vi "Swerve_Module Drive Read Config.vi"(6 "Send Cmd Timout(ms)":u32=300, 8 "Error":errorcluster, 10 "Module Drive Config Data":T1={"ModuleDrive Ver"=0, "Output"={"Type"=enum."Counter-Clockwise", "Neutral"=enum."EEPROMSetting", "Max"={"FWD"=0.0, "REV"=0.04}, "Min"={"FWD"=0.0, "REV"=0.0}, "OL Ramp Rate (S)"=0.0, "Dead Band"=0.0}, "CL"={"Gains"={"P"=1.0, "I"=0.01, "D"=0.0, "F"=0.0}, "Error Allowed"={"High"=0.0, "Low"=0.0}, "I Zone"={"High"=10000.0, "Low"=-1000.0}, "Max Out"={"FWD"=1.0, "REV"=-1.0}, "Max I Accu"={"High"=10.0, "Low"=-10.0}, "CL Ramp Rate (S)"=0.0}, "VoltageComp"={"Enable"=FALSE, "Value"=0.0}} {"Output"."Min"."REV" format="%.2f"; "Output"."Min"."FWD" format="%.2f"; "Output"."Max"."REV" format="%.2f"; "Output"."Max"."FWD" format="%.2f"; "VoltageComp"."Value" format="%.1g"; "CL"."Max I Accu"."Low" format="%#.8f"; "CL"."Max I Accu"."High" format="%#.8f"; "CL"."Gains"."F" format="%#.8f"; "CL"."Gains"."D" format="%#.8f"; "CL"."Gains"."I" format="%#.8f"; "CL"."Gains"."P" format="%#.8f"; "CL"."Error Allowed"."Low" format="%#.8f"; "CL"."Error Allowed"."High" format="%#.8f"; "CL"."I Zone"."Low" format="%#.8f"; "CL"."I Zone"."High" format="%#.8f"; "CL"."Max Out"."REV" format="%.2f"; "CL"."Max Out"."FWD" format="%.2f"}, 11 "PhoenixMotorControlDevRef":T10={"DeviceStatus"={"status"=FALSE, "code"=0, "source"=""}, "Type"=enum."PWM", "PWM"={"PWM Channel"=enum."Invalid", "DeadBand"={"Name"="", "maxPositivePwm"=0, "minPositivePwm"=0, "centerPwm"=0, "maxNegativePwm"=0, "minNegativePwm"=0, "angularRange"=0}}, "CAN"={"Device Number"=0, "SetOutput VI Ref"=variant, "GetOutput VI Ref"=variant, "Enable VI Ref"=variant, "Disable VI Ref"=variant, "Data"=variant}, "Invert"=FALSE, "DIO PWM"={"PWM \"Enable\" Channel"=enum."Invalid", "DIOChannel"=enum."Invalid", "PWM Rate"=0.0}}) -> (0 "Error Out":errorcluster, 2 "Module Azimuth Config Data Out":T1={"ModuleDrive Ver"=0, "Output"={"Type"=enum."Counter-Clockwise", "Neutral"=enum."EEPROMSetting", "Max"={"FWD"=0.0, "REV"=0.04}, "Min"={"FWD"=0.0, "REV"=0.0}, "OL Ramp Rate (S)"=0.0, "Dead Band"=0.0}, "CL"={"Gains"={"P"=1.0, "I"=0.01, "D"=0.0, "F"=0.0}, "Error Allowed"={"High"=0.0, "Low"=0.0}, "I Zone"={"High"=10000.0, "Low"=-1000.0}, "Max Out"={"FWD"=1.0, "REV"=-1.0}, "Max I Accu"={"High"=10.0, "Low"=-10.0}, "CL Ramp Rate (S)"=0.0}, "VoltageComp"={"Enable"=FALSE, "Value"=0.0}} {"Output"."Min"."REV" format="%.2f"; "Output"."Min"."FWD" format="%.2f"; "Output"."Max"."REV" format="%.2f"; "Output"."Max"."FWD" format="%.2f"; "VoltageComp"."Value" format="%.1g"; "CL"."Max I Accu"."Low" format="%#.8f"; "CL"."Max I Accu"."High" format="%#.8f"; "CL"."Gains"."F" format="%#.8f"; "CL"."Gains"."D" format="%#.8f"; "CL"."Gains"."I" format="%#.8f"; "CL"."Gains"."P" format="%#.8f"; "CL"."Error Allowed"."Low" format="%#.8f"; "CL"."Error Allowed"."High" format="%#.8f"; "CL"."I Zone"."Low" format="%#.8f"; "CL"."I Zone"."High" format="%#.8f"; "CL"."Max Out"."REV" format="%.2f"; "CL"."Max Out"."FWD" format="%.2f"}, 3 "Module Azimuth Ref Out":T10)   [LabVIEW 2023]
uses:
  <vilib>/Utility/Data Type/NI_Data Type.lvlib
  <vilib>/Rock Robotics/WPI/ThirdParty/Phoenix-LabVIEW/Motor Controller/Controls/CTRE_Phoenix_MotorControl_RemoteSourceType.ctl
  <vilib>/Rock Robotics/WPI/ThirdParty/Phoenix-LabVIEW/Motor Controller/Controls/CTRE_Phoenix_MotorControl_FeedbackDevice_TalonFX.ctl
  <vilib>/Rock Robotics/WPI/ThirdParty/Phoenix-LabVIEW/Motor Controller/Controls/CTRE_Phoenix_MotorControl_NeutralMode.ctl
  <vilib>/Rock Robotics/WPI/ThirdParty/Phoenix-LabVIEW/Motor Controller/Controls/CTRE_Phoenix_MotorControl_VelocityMeasurementPeriod.ctl
  <vilib>/Rock Robotics/WPI/ThirdParty/Phoenix-LabVIEW/Motor Controller/Controls/CTRE_Phoenix_MotorControl_SlotStructure.ctl
  <vilib>/Rock Robotics/WPI/ThirdParty/Phoenix-LabVIEW/Motor Controller/Controls/CTRE_Phoenix_MotorControl_FilterStruct.ctl
  <vilib>/Rock Robotics/WPI/ThirdParty/Phoenix-LabVIEW/Controls/CTRE_Phoenix_CustomParamConfiguration.ctl
  <vilib>/Rock Robotics/WPI/ThirdParty/Phoenix-LabVIEW/Motor Controller/Controls/CTRE_Phoenix_MotorControl_BaseConfigurables.ctl
  <vilib>/Rock Robotics/WPI/ThirdParty/Phoenix-LabVIEW/Motor Controller/Controls/CTRE_Phoenix_MotorControl_LimitSwitchNormal.ctl
  <vilib>/Rock Robotics/WPI/ThirdParty/Phoenix-LabVIEW/Motor Controller/Controls/CTRE_Phoenix_MotorControl_LimitSwitchSource_Local.ctl
  <vilib>/Rock Robotics/WPI/ThirdParty/Phoenix-LabVIEW/Motor Controller/Controls/CTRE_Phoenix_MotorControl_SupplyCurrentLimitConfiguration.ctl
  <vilib>/Rock Robotics/WPI/ThirdParty/Phoenix-LabVIEW/Motor Controller/Controls/CTRE_Phoenix_MotorControl_StatorCurrentLimitConfiguration.ctl
  <vilib>/Rock Robotics/WPI/ThirdParty/Phoenix-LabVIEW/Motor Controller/Controls/CTRE_Phoenix_MotorControl_MotorCommutation_TalonFX.ctl
  <vilib>/Rock Robotics/WPI/ThirdParty/Phoenix-LabVIEW/CANCoder/Controls/CTRE_Phoenix_CANcoder_AbsoluteSensorRange.ctl
  <vilib>/Rock Robotics/WPI/ThirdParty/Phoenix-LabVIEW/CANCoder/Controls/CTRE_Phoenix_CANcoder_SensorInitializationStrategy.ctl
  <vilib>/Rock Robotics/WPI/ThirdParty/Phoenix-LabVIEW/Motor Controller/Controls/CTRE_Phoenix_MotorControl_TalonFXMotorControllerConfigurables.ctl
  <vilib>/Rock Robotics/WPI/ThirdParty/Phoenix-LabVIEW/Motor Controller/Controls/CTRE_Phoenix_MotorControl_TalonFXInvertType.ctl
  <vilib>/Rock Robotics/SystemInterfaces/DIO/FPGA_DIOPWMChannel.ctl
  <vilib>/Rock Robotics/WPI/PWM/WPI_PWMDeadband.ctl
  <vilib>/Rock Robotics/WPI/MotorControl/WPI_MotorControlType.ctl
  <vilib>/Rock Robotics/SystemInterfaces/DIO/FPGA_DIOChannel.ctl
  <vilib>/Rock Robotics/WPI/MotorControl/WPI_MotorControlDeviceRef.ctl
  Shared Code/TypeDefs/Cluster_High-Low.ctl
  Shared Code/TypeDefs/Cluster_PID Gains.ctl
  Shared Code/TypeDefs/Cluster_PID Config.ctl
  Shared Code/TypeDefs/Cluster_Enable-Value DBL.ctl
  Shared Code/TypeDefs/Cluster_Swerve Module Drive Config Data.ctl
  Shared Code/TypeDefs/Cluster_FWD  REV Values.ctl
  Shared Code/TypeDefs/Cluster_Config Motor Output.ctl
panel:
  # "Tune to Output\nto 1023 Max"
  # "Tune to Output\nto 1023 Max"
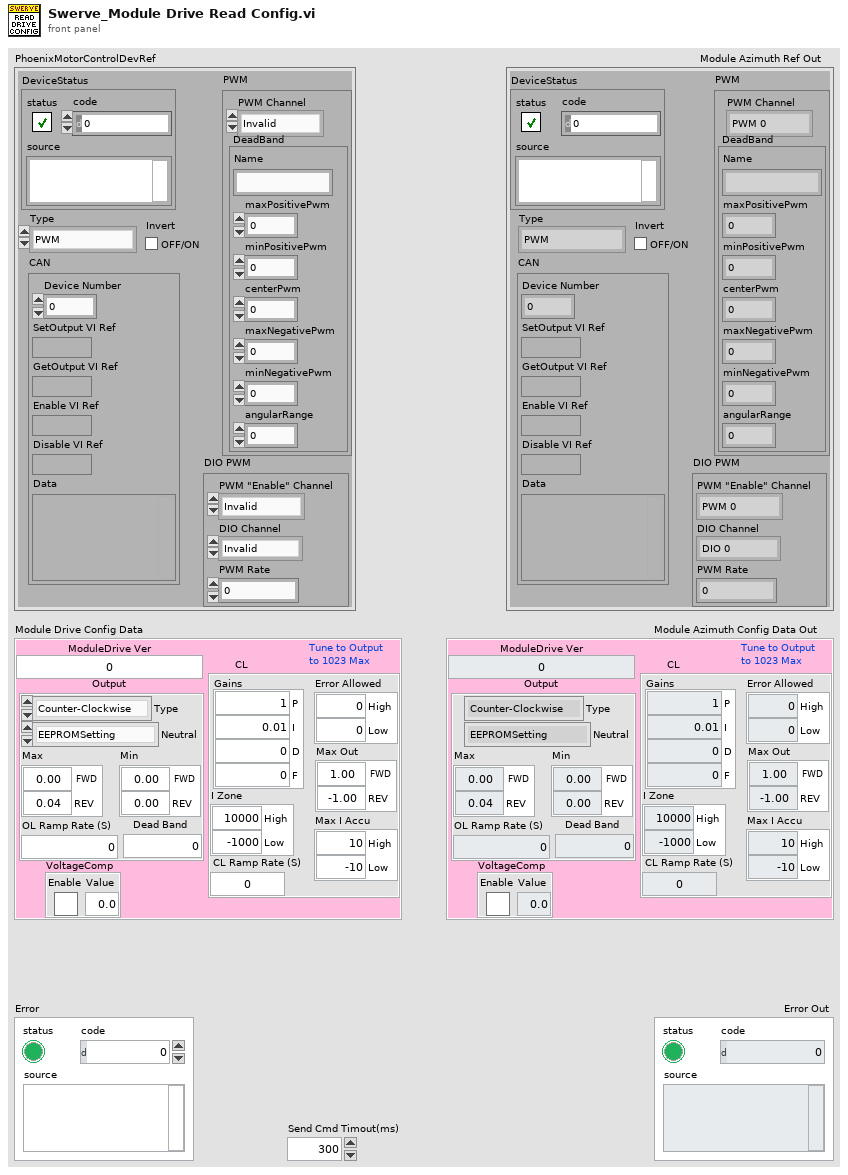
[diagram p1: front panel]
types:
  T1 = typedef "Cluster_Swerve Module Drive Config Data.ctl" = cluster{"ModuleDrive Ver":u64, "Output":T2, "CL":T6, "VoltageComp":T9}
  T2 = typedef "Cluster_Config Motor Output.ctl" = cluster{"Type":T3, "Neutral":T4, "Max":T5, "Min":T5, "OL Ramp Rate (S)":dbl, "Dead Band":dbl}
  T3 = typedef "CTRE_Phoenix_MotorControl_TalonFXInvertType.ctl" = enum16{"Counter-Clockwise", "Clockwise"}
  T4 = typedef "CTRE_Phoenix_MotorControl_NeutralMode.ctl" = enum8{"EEPROMSetting", "Override to Coast", "Override to Brake"}
  T5 = typedef "Cluster_FWD  REV Values.ctl" = cluster{"FWD":dbl, "REV":dbl}
  T6 = typedef "Cluster_PID Config.ctl" = cluster{"Gains":T7, "Error Allowed":T8, "I Zone":T8, "Max Out":T5, "Max I Accu":T8, "CL Ramp Rate (S)":dbl}
  T7 = typedef "Cluster_PID Gains.ctl" = cluster{"P":dbl, "I":dbl, "D":dbl, "F":dbl}
  T8 = typedef "Cluster_High-Low.ctl" = cluster{"High":dbl, "Low":dbl}
  T9 = typedef "Cluster_Enable-Value DBL.ctl" = cluster{"Enable":bool, "Value":dbl}
  T10 = typedef "WPI_MotorControlDeviceRef.ctl" = cluster{"DeviceStatus":errorcluster, "Type":T11, "PWM":cluster{"PWM Channel":T12, "DeadBand":T13}, "CAN":cluster{"Device Number":u8, "SetOutput VI Ref":variant, "GetOutput VI Ref":variant, "Enable VI Ref":variant, "Disable VI Ref":variant, "Data":variant}, "Invert":bool, "DIO PWM":cluster{"PWM \"Enable\" Channel":T12, "DIOChannel":T14, "PWM Rate":dbl}}
  T11 = typedef "WPI_MotorControlType.ctl" = enum16{"PWM", "CAN", "DIO PWM"}
  T12 = typedef "FPGA_DIOPWMChannel.ctl" = enum8{"PWM 0", "PWM 1", "PWM 2", "PWM 3", "PWM 4", "PWM 5", "PWM 6", "PWM 7", "PWM 8", "PWM 9", "PWM MXP 0", "PWM MXP 1", "PWM MXP 2", "PWM MXP 3", "PWM MXP 4", "PWM MXP 5", "PWM MXP 6", "PWM MXP 7", "PWM MXP 8", "PWM MXP 9", "Invalid"}
  T13 = typedef "WPI_PWMDeadband.ctl" = cluster{"Name":string, "maxPositivePwm":i32, "minPositivePwm":i32, "centerPwm":i32, "maxNegativePwm":i32, "minNegativePwm":i32, "angularRange":u16}
  T14 = typedef "FPGA_DIOChannel.ctl" = enum8{"DIO 0", "DIO 1", "DIO 2", "DIO 3", "DIO 4", "DIO 5", "DIO 6", "DIO 7", "DIO 8", "DIO 9", "DIO MXP 0", "DIO MXP 1", "DIO MXP 2", "DIO MXP 3", "DIO MXP 4", "DIO MXP 5", "DIO MXP 6", "DIO MXP 7", "DIO MXP 8", "DIO MXP 9", "DIO MXP 10", "DIO MXP 11", "DIO MXP 12", "DIO MXP 13", "DIO MXP 14", "DIO MXP 15", "SPI Port CS1", "SPI Port CS2", "SPI Port CS3", "SPI Port MISO", "SPI Port MOSI", "Invalid"}
  T15 = typedef "CTRE_Phoenix_MotorControl_TalonFXMotorControllerConfigurables.ctl" = cluster{"Base Configurables":T16, "primaryPID":cluster{"selectedFeedbackCoefficient":dbl, "selectedFeedbackSensor":T22}, "auxiliaryPID":cluster{"selectedFeedbackCoefficient":dbl, "selectedFeedbackSensor":T22}, "forwardLimitSwitchNormal":T23, "reverseLimitSwitchNormal":T23, "forwardLimitSwitchDeviceID":i32, "reverseLimitSwitchDeviceID":i32, "forwardLimitSwitchSource":T24, "reverseLimitSwitchSource":T24, "sum0Term":T22, "sum1Term":T22, "diff0Term":T22, "diff1Term":T22, "Supply Current Limit Configuration":T25, "Stator Current Limit Configuration":T26, "Motor Commutation":T27, "Absolute Sensor Range":T28, "Integrated Sensor Offset (Degrees)":dbl, "Sensor Initialization Strategy":T29}
  T16 = typedef "CTRE_Phoenix_MotorControl_BaseConfigurables.ctl" = cluster{"openLoopRamp":dbl, "closedLoopRamp":dbl, "peakOutputForward":dbl, "peakOutputReverse":dbl, "nominalOutputForward":dbl, "nominalOutputReverse":dbl, "neutralDeadband":dbl, "voltageCompSaturation":dbl, "voltageMeasurementFilter":i32, "velocityMeasurementPeriod":T17, "velocityMeasurementWindow":i32, "forwardSoftLimitThreshold":i32, "reverseSoftLimitThreshold":i32, "forwardSoftLimitEnable":bool, "reverseSoftLimitEnable":bool, "slot0":T18, "slot1":T18, "slot2":T18, "slot3":T18, "auxPIDPolarity":bool, "remoteFilter0":T19, "remoteFilter1":T19, "motionCruiseVelocity":i32, "motionAcceleration":i32, "motionProfileTrajectoryPeriod":i32, "feedbackNotContinuous":bool, "remoteSensorClosedLoopDisableNeutralOnLOS":bool, "clearPositionOnLimitF":bool, "clearPositionOnLimitR":bool, "clearPositionOnQuadIdx":bool, "limitSwitchDisableNeutralOnLOS":bool, "softLimitDisableNeutralOnLOS":bool, "pulseWidthPeriod_EdgesPerRot":i32, "pulseWidthPeriod_FilterWindowSz":i32, "customParam":T21, "trajectoryInterpolationEnable":bool}
  T17 = typedef "CTRE_Phoenix_MotorControl_VelocityMeasurementPeriod.ctl" = u16
  T18 = typedef "CTRE_Phoenix_MotorControl_SlotStructure.ctl" = cluster{"P":dbl, "I":dbl, "D":dbl, "F":dbl, "integralZone":dbl, "allowableClosedLoopError":i32, "maxIntegralAccumulator":dbl, "closedLoopPeakOutput":dbl, "closedLoopPeriod":i32}
  T19 = typedef "CTRE_Phoenix_MotorControl_FilterStruct.ctl" = cluster{"remoteSensorDeviceID":u8, "remoteSensorSource":T20}
  T20 = typedef "CTRE_Phoenix_MotorControl_RemoteSourceType.ctl" = enum16{"Off", "Talon SRX Selected Sensor", "Pigeon IMU Yaw", "Pigeon IMU Pitch", "Pigeon IMU Roll", "CANifier Quadrature", "CANifier PWM Input 0", "CANifier PWM Input 1", "CANifier PWM Input 2", "CANifier PWM Input 3", "Gadgeteer Pigeon Yaw", "Gadgeteer Pigeon Pitch", "Gadgeteer Pigeon Roll", "CANCoder"}
  T21 = typedef "CTRE_Phoenix_CustomParamConfiguration.ctl" = cluster{"customParam0":i32, "customParam1":i32}
  T22 = typedef "CTRE_Phoenix_MotorControl_FeedbackDevice_TalonFX.ctl" = i8
  T23 = typedef "CTRE_Phoenix_MotorControl_LimitSwitchNormal.ctl" = enum16{"Normally Open", "Normally Closed", "Disabled"}
  T24 = typedef "CTRE_Phoenix_MotorControl_LimitSwitchSource_Local.ctl" = enum16{"Feedback Connector", "Remote Talon SRX", "Remote CANifier", "Deactivated"}
  T25 = typedef "CTRE_Phoenix_MotorControl_SupplyCurrentLimitConfiguration.ctl" = cluster{"Enable?":bool, "Current Limit":dbl, "Threshold Current":dbl, "Threshold Time":dbl}
  T26 = typedef "CTRE_Phoenix_MotorControl_StatorCurrentLimitConfiguration.ctl" = cluster{"Enable?":bool, "Current Limit":dbl, "Threshold Current":dbl, "Threshold Time":dbl}
  T27 = typedef "CTRE_Phoenix_MotorControl_MotorCommutation_TalonFX.ctl" = enum16{"Trapezoidal"}
  T28 = typedef "CTRE_Phoenix_CANcoder_AbsoluteSensorRange.ctl" = enum16{"Unsigned [0 to 360)", "Signed [-180 to +180)"}
  T29 = typedef "CTRE_Phoenix_CANcoder_SensorInitializationStrategy.ctl" = enum16{"Boot To Zero", "Boot To Absolute Position"}
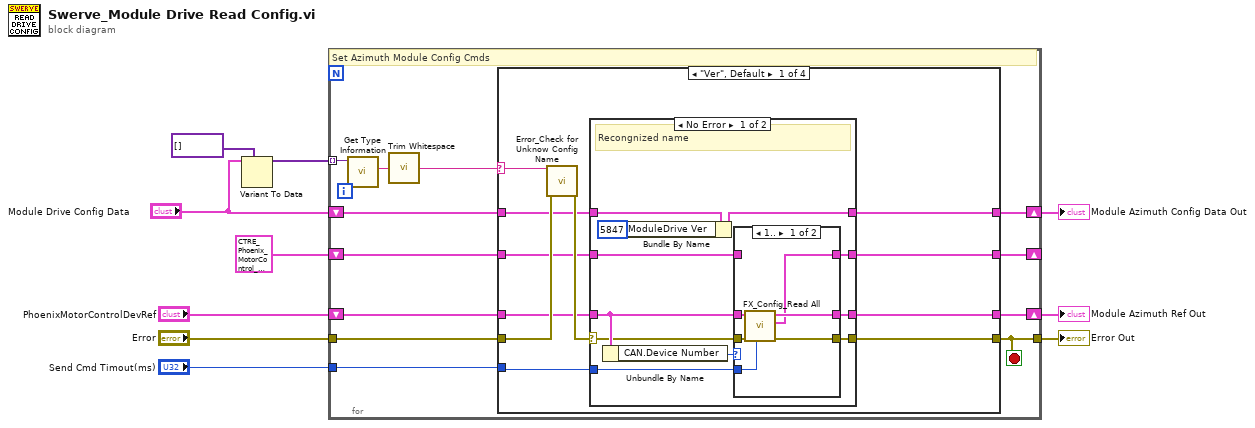
[diagram p0: block diagram]
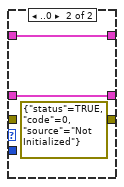
[diagram p2: hidden frame]
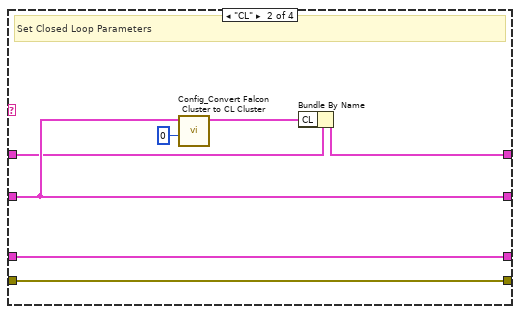
[diagram p4: hidden frame]
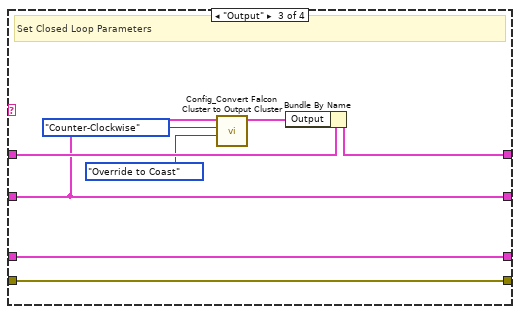
[diagram p5: hidden frame]
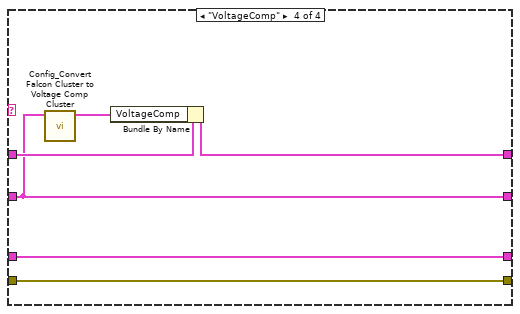
[diagram p6: hidden frame]
diagram:
  n1 = Variant To Data(type=variant[] [], Variant="Module Drive Config Data") -> (data=w1:variant[])  [unwired: 1 in, 1 out]
  n2 = for {
    tunnel: "Send Cmd Timout(ms)" -> [w21]
    shift-right: [w22] -> w10
    shift-left: "PhoenixMotorControlDevRef" -> [w19]
    tunnel: w1 -> [w18] mode=indexing
    tunnel: "Error" -> [w11]
    tunnel: [w16] -> w9
    shift-right: [w17] -> w3
    shift-left: "Module Drive Config Data" -> [w20]
    shift-right: [w15] -> _
    shift-left: T15 {"Base Configurables"={"openLoopRamp"=0.0, "closedLoopRamp"=0.0, "peakOutputForward"=1.0, "peakOutputReverse"=-1.0, "nominalOutputForward"=0.0, "nominalOutputReverse"=0.0, "neutralDeadband"=0.04, "voltageCompSaturation"=0.0, "voltageMeasurementFilter"=32, "velocityMeasurementPeriod"=100, "velocityMeasurementWindow"=64, "forwardSoftLimitThreshold"=0, "reverseSoftLimitThreshold"=0, "forwardSoftLimitEnable"=FALSE, "reverseSoftLimitEnable"=FALSE, "slot0"={"P"=0.0, "I"=0.0, "D"=0.0, "F"=0.0, "integralZone"=0.0, "allowableClosedLoopError"=0, "maxIntegralAccumulator"=0.0, "closedLoopPeakOutput"=1.0, "closedLoopPeriod"=1}, "slot1"={"P"=0.0, "I"=0.0, "D"=0.0, "F"=0.0, "integralZone"=0.0, "allowableClosedLoopError"=0, "maxIntegralAccumulator"=0.0, "closedLoopPeakOutput"=1.0, "closedLoopPeriod"=1}, "slot2"={"P"=0.0, "I"=0.0, "D"=0.0, "F"=0.0, "integralZone"=0.0, "allowableClosedLoopError"=0, "maxIntegralAccumulator"=0.0, "closedLoopPeakOutput"=1.0, "closedLoopPeriod"=1}, "slot3"={"P"=0.0, "I"=0.0, "D"=0.0, "F"=0.0, "integralZone"=0.0, "allowableClosedLoopError"=0, "maxIntegralAccumulator"=0.0, "closedLoopPeakOutput"=1.0, "closedLoopPeriod"=1}, "auxPIDPolarity"=FALSE, "remoteFilter0"={"remoteSensorDeviceID"=0, "remoteSensorSource"=enum."Off"}, "remoteFilter1"={"remoteSensorDeviceID"=0, "remoteSensorSource"=enum."Off"}, "motionCruiseVelocity"=0, "motionAcceleration"=0, "motionProfileTrajectoryPeriod"=0, "feedbackNotContinuous"=FALSE, "remoteSensorClosedLoopDisableNeutralOnLOS"=FALSE, "clearPositionOnLimitF"=FALSE, "clearPositionOnLimitR"=FALSE, "clearPositionOnQuadIdx"=FALSE, "limitSwitchDisableNeutralOnLOS"=FALSE, "softLimitDisableNeutralOnLOS"=FALSE, "pulseWidthPeriod_EdgesPerRot"=1, "pulseWidthPeriod_FilterWindowSz"=1, "customParam"={"customParam0"=0, "customParam1"=0}, "trajectoryInterpolationEnable"=TRUE}, "primaryPID"={"selectedFeedbackCoefficient"=1.0, "selectedFeedbackSensor"=1}, "auxiliaryPID"={"selectedFeedbackCoefficient"=1.0, "selectedFeedbackSensor"=1}, "forwardLimitSwitchNormal"=enum."Normally Open", "reverseLimitSwitchNormal"=enum."Normally Open", "forwardLimitSwitchDeviceID"=0, "reverseLimitSwitchDeviceID"=0, "forwardLimitSwitchSource"=enum."Feedback Connector", "reverseLimitSwitchSource"=enum."Feedback Connector", "sum0Term"=1, "sum1Term"=1, "diff0Term"=1, "diff1Term"=1, "Supply Current Limit Configuration"={"Enable?"=FALSE, "Current Limit"=0.0, "Threshold Current"=0.0, "Threshold Time"=0.0}, "Stator Current Limit Configuration"={"Enable?"=FALSE, "Current Limit"=0.0, "Threshold Current"=0.0, "Threshold Time"=0.0}, "Motor Commutation"=enum."Trapezoidal", "Absolute Sensor Range"=enum."Unsigned [0 to 360)", "Integrated Sensor Offset (Degrees)"=0.0, "Sensor Initialization Strategy"=enum."Boot To Zero"} ("Talon FX Configurables") -> [w14]
    stop <- w16 stop-if-true
    # "Set Azimuth Module Config Cmds"
    n3 = call <vilib>:"Get Type Information.vi"("variant"=w18) -> ("name"=w13:string)  [unwired: 6 in, 4 out]
    n4 = call <vilib>:"Trim Whitespace.vi"("string"=w13) -> ("trimmed string"=w12:string)  [unwired: 1 in]
    n5 = case shown="\"Ver\", Default" w12 {
      selector: w12 -> [w28 _ _ _]
      tunnel: [w31 w63 w71 w76] -> w16
      tunnel: w21 -> [w23 _ _ _]
      tunnel: w19 -> [w25 w64 w72 w75]
      tunnel: [w24 w64 w72 w75] -> w22
      tunnel: w20 -> [w30 w60 w70 w77]
      tunnel: [w27 w58 w68 w78] -> w17
      tunnel: [w26 w62 w67 w73] -> w15
      tunnel: w14 -> [w29 w62 w67 w73]
      tunnel: w11 -> [w32 w63 w71 w76]
      frame "Ver", Default {
        n6 = call "Error_Check for Unknow Config Name.vi"("error in (no error)"=w32, "Config Name"=w28) -> ("error out"=w33:errorcluster)  [unwired: 9 in]
        n7 = case shown="No Error" w33 {
          selector: w33 -> [w34 w55]
          tunnel: [w43 w55] -> w31
          tunnel: w25 -> [w42 w54]
          tunnel: [w41 w54] -> w24
          tunnel: [w40 w56] -> w26
          tunnel: w23 -> [w39 _]
          tunnel: w29 -> [w38 w56]
          tunnel: [w36 w57] -> w27
          tunnel: w30 -> [w35 w57]
          frame No Error {
            # "Recongnized name"
            n8 = Unbundle By Name(w42) -> ("CAN.Device Number"=w44:u8)
            n9 = Bundle By Name(cluster=w35, "ModuleDrive Ver"=u64 5847 ("ModuleAzimuth Ver")) -> (w36:T1)
            n10 = case shown="1.." w44 {
              tunnel: [w48 errorcluster {"status"=TRUE, "code"=0, "source"="Not Initialized"} ("error out")] -> w43
              tunnel: w42 -> [w50 w52]
              tunnel: [w47 w52] -> w41
              tunnel: [w46 w51] -> w40
              tunnel: w34 -> [w49 _]
              tunnel: w39 -> [w45 _]
              tunnel: w38 -> [_ w51]
              frame 1.. {
                n11 = call "FX_Config_Read All.vi"("Send Cmd Timout(ms)"=w45, "Error"=w49, "PhoenixMotorControlDevRef"=w50) -> ("Error Out"=w48:errorcluster, "FX Config Out"=w46:T15, "Ref Out"=w47:T10)  [unwired: 6 in]
              }
              frame ..0 {
              }
            }
          }
          frame Error {
            # "Unrecognized name"
          }
        }
      }
      frame "CL" {
        # "Set Closed Loop Parameters"
        n12 = call "Config_Convert Falcon Cluster to CL Cluster.vi"("Slot"=0, "Talon FX Configurables"=w62) -> ("CL"=w59:T6)  [unwired: 8 in, 1 out]
        n13 = Bundle By Name(cluster=w60, "CL"=w59) -> (w58:T1)
      }
      frame "Output" {
        # "Set Closed Loop Parameters"
        n14 = call "Config_Convert Falcon Cluster to Output Cluster.vi"("Neutral Mode"=CTRE_Phoenix_MotorControl_NeutralMode."Override to Coast", "Rotation Type"=CTRE_Phoenix_MotorControl_TalonFXInvertType."Counter-Clockwise", "Talon FX Configurables"=w67) -> ("Motor Output Out"=w69:T2)  [unwired: 8 in]
        n15 = Bundle By Name(cluster=w70, "Output"=w69) -> (w68:T1)
      }
      frame "VoltageComp" {
        n16 = call "Config_Convert Falcon Cluster to Voltage Comp Cluster.vi"("Talon FX Configurables"=w73) -> ("VoltageComp"=w74:T9)  [unwired: 10 in]
        n17 = Bundle By Name(cluster=w77, "VoltageComp"=w74) -> (w78:T1)
      }
    }
  }
  "Module Azimuth Ref Out" <- w10
  "Error Out" <- w9
  "Module Azimuth Config Data Out" <- w3
